vi "Prepare Controls.vi"(8 "error in (no error)":errorcluster, 11 "ValveControlModule in":refnum<class "ValveControlModule.lvclass">) -> (0 "error out":errorcluster, 3 "ValveControlModule out":refnum<class "ValveControlModule.lvclass">)   [LabVIEW 2020, in "VolatusControl.lvlib" / "ValveControlModule.lvclass"]
uses:
  ValveControlModule.lvclass
  ValveControlModule.lvclass/ValveControlModule.ctl
  Volatus/Module/Module.lvclass
  Valve/ValveControl.lvclass
  C:/dev/lv20CE/relink/lv-volatus/Volatus/Module/Module.lvclass
  C:/dev/lv20CE/relink/lv-volatus/VolatusControl/ValveControlModule/ValveControlModule.lvclass
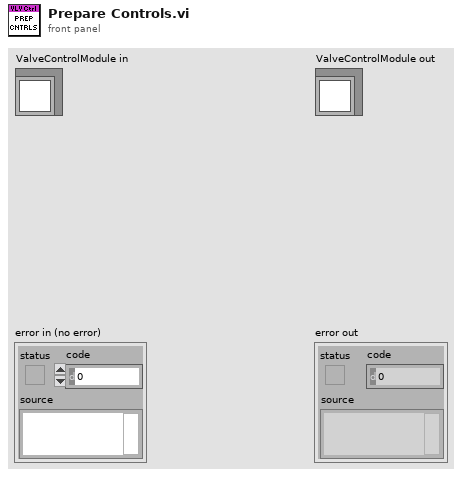
[diagram p1: front panel]
types:
  T1 = map{string, refnum<class "ValveControl.lvclass">}
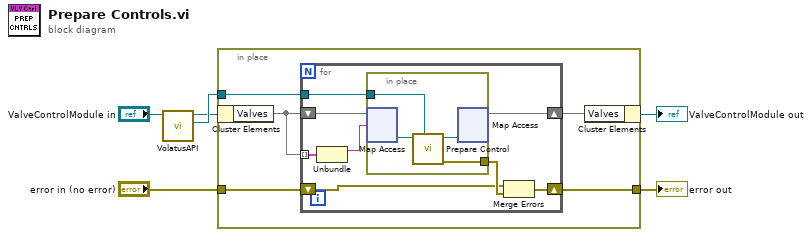
[diagram p0: block diagram]
diagram:
  n1 = call "VolatusAPI.vi"("Module in"="ValveControlModule in") -> ("VolatusAPI"=w5:refnum<class "VolatusAPI.lvclass">, "Module out"=w4:refnum<class "ValveControlModule.lvclass">)  [unwired: 9 in]
  n2 = in-place {
    in-place-border: w5 -> [w10]
    in-place-border: [w8] -> w2
    in-place-border: "error in (no error)" -> [w7]
    n3 = in-place-cluster #1(w4) -> ("Valves"=w11:T1)
    n4 = for {
      shift-right: [w15] -> w9
      shift-left: w11 -> [w18]
      tunnel: w11 -> [w19] mode=indexing
      tunnel: w10 -> [w16]
      shift-right: [w13] -> w8
      shift-left: w7 -> [w12]
      n5 = Unbundle(w19) -> ("Name"=w17:string)  [unwired: 1 out]
      n6 = in-place {
        in-place-border: w16 -> [w22]
        in-place-border: [w20] -> w14
        n7 = in-place-map #2(w18, w17) -> (w23:refnum<class "ValveControl.lvclass">)  [unwired: 1 in, 1 out]
        n8 = call-dynamic "Prepare Control.vi"("VolatusAPI"=w22, "ValveControl in"=w23) -> ("error out"=w20:errorcluster, "ValveControl out"=w21:refnum<class "ValveControl.lvclass">)  [unwired: 8 in]
        n9 = in-place-map #2(w21) -> (w15:T1)  [unwired: 1 in, 2 out]
      }
      n10 = Merge Errors(w12, w14) -> (w13:errorcluster)
    }
    n11 = in-place-cluster #1("Valves"=w9) -> (→"ValveControlModule out":refnum<class "ValveControlModule.lvclass">)
  }
  "error out" <- w2
